vi "Build-timeline.vi"(8 "error in (no error)":errorcluster, 10 "Temp-timeline in":T1={"Previous point"={"Start time [µs]"=0, "End time [µs]"=0, "X [mm]"=0.0, "Y [mm]"=0.0, "Type"=enum."BeginJob", "Speed [mm/µs]"=0.0, "Direction [rad]"=0.0, "X [bit]"=0, "Y [bit]"=0, "Speed [bit/µs]"=0.0, "Power [W]"=0.0, "Power [bit]"=0, "JumpDelay"=0, "MarkDelay"=0, "PolyDelay"=0, "LaserOnDelay"=0, "LaserOffDelay"=0, "LaserPowerDelay"=0, "LaserEnableDelay"=0, "Xraw [mm]"=0.0, "Yraw [mm]"=0.0}, "Current point"={"Start time [µs]"=0, "End time [µs]"=0, "X [mm]"=0.0, "Y [mm]"=0.0, "Type"=enum."BeginJob", "Speed [mm/µs]"=0.0, "Direction [rad]"=0.0, "X [bit]"=0, "Y [bit]"=0, "Speed [bit/µs]"=0.0, "Power [W]"=0.0, "Power [bit]"=0, "JumpDelay"=0, "MarkDelay"=0, "PolyDelay"=0, "LaserOnDelay"=0, "LaserOffDelay"=0, "LaserPowerDelay"=0, "LaserEnableDelay"=0, "Xraw [mm]"=0.0, "Yraw [mm]"=0.0}, "Path"=[], "Current properties"={"ItemID"=0, "Start time"=0, "EffectiveOffset"=[0.0, 0.0], "EffectiveTranfsorm"=[[1.0, 0.0], [0.0, 1.0]], "Z-Offset"=0.0, "Units"=enum."mm", "LaserPower"=0, "Started"=FALSE, "Enabled"=FALSE, "FieldOffset"=[0.0, 0.0], "Offset"=[0.0, 0.0], "TransformEnable"=TRUE, "XYCalFactor"=196.0, "JumpSpeed"={"unit/us"=0.0, "Tick interval us"=0, "Bits per interval"=0}, "MarkSpeed"={"unit/us"=0.0, "Tick interval us"=0, "Bits per interval"=0}}}, 11 "Element-XML in":refnum<class "BeginJob.lvclass">) -> (0 "error out":errorcluster, 2 "Temp-timeline":T1={"Previous point"={"Start time [µs]"=0, "End time [µs]"=0, "X [mm]"=0.0, "Y [mm]"=0.0, "Type"=enum."BeginJob", "Speed [mm/µs]"=0.0, "Direction [rad]"=0.0, "X [bit]"=0, "Y [bit]"=0, "Speed [bit/µs]"=0.0, "Power [W]"=0.0, "Power [bit]"=0, "JumpDelay"=0, "MarkDelay"=0, "PolyDelay"=0, "LaserOnDelay"=0, "LaserOffDelay"=0, "LaserPowerDelay"=0, "LaserEnableDelay"=0, "Xraw [mm]"=0.0, "Yraw [mm]"=0.0}, "Current point"={"Start time [µs]"=0, "End time [µs]"=0, "X [mm]"=0.0, "Y [mm]"=0.0, "Type"=enum."BeginJob", "Speed [mm/µs]"=0.0, "Direction [rad]"=0.0, "X [bit]"=0, "Y [bit]"=0, "Speed [bit/µs]"=0.0, "Power [W]"=0.0, "Power [bit]"=0, "JumpDelay"=0, "MarkDelay"=0, "PolyDelay"=0, "LaserOnDelay"=0, "LaserOffDelay"=0, "LaserPowerDelay"=0, "LaserEnableDelay"=0, "Xraw [mm]"=0.0, "Yraw [mm]"=0.0}, "Path"=[], "Current properties"={"ItemID"=0, "Start time"=0, "EffectiveOffset"=[0.0, 0.0], "EffectiveTranfsorm"=[[1.0, 0.0], [0.0, 1.0]], "Z-Offset"=0.0, "Units"=enum."mm", "LaserPower"=0, "Started"=FALSE, "Enabled"=FALSE, "FieldOffset"=[0.0, 0.0], "Offset"=[0.0, 0.0], "TransformEnable"=TRUE, "XYCalFactor"=196.0, "JumpSpeed"={"unit/us"=0.0, "Tick interval us"=0, "Bits per interval"=0}, "MarkSpeed"={"unit/us"=0.0, "Tick interval us"=0, "Bits per interval"=0}}}, 3 "Element-XML out":refnum<class "BeginJob.lvclass">)   [LabVIEW 2013, in "MaterialCharacterization.lvlib" / "BeginJob.lvclass"]
uses:
  BeginJob.lvclass
  ScanParser/Path-buffer.ctl
  ScanParser/Point-buffer.ctl
  Elements.ctl
  ScanParser/Property-buffer.ctl
  ScanParser/Units.ctl
  ScanParser/Speed.ctl
  Element-XML.lvclass
  ScanParser/MC-ScanParser.lvclass
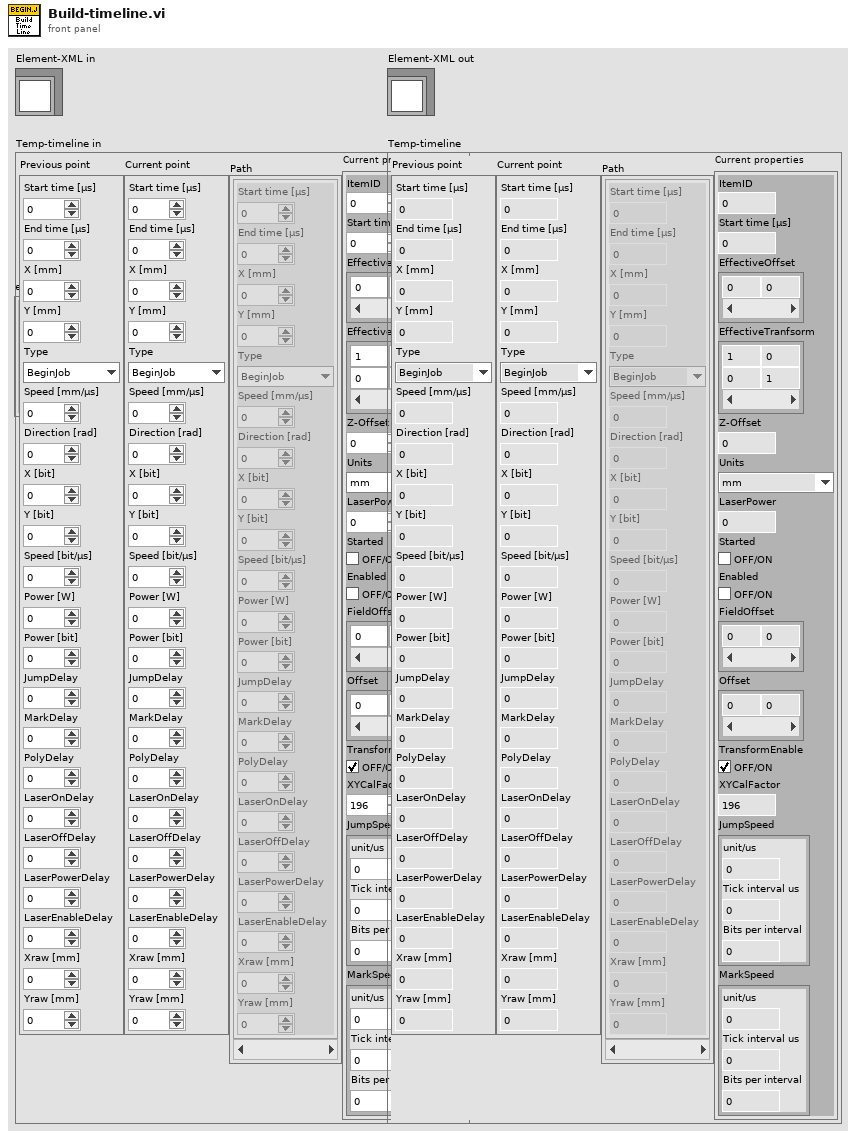
[diagram p1: front panel]
types:
  T1 = typedef "MaterialCharacterization.lvlib/MC-ScanParser.lvclass/Path-buffer.ctl" = cluster{"Previous point":T2, "Current point":T2, "Path":T2[], "Current properties":T4}
  T2 = typedef "MaterialCharacterization.lvlib/MC-ScanParser.lvclass/Point-buffer.ctl" = cluster{"Start time [µs]":i64, "End time [µs]":i64, "X [mm]":dbl, "Y [mm]":dbl, "Type":T3, "Speed [mm/µs]":dbl, "Direction [rad]":dbl, "X [bit]":i16, "Y [bit]":i16, "Speed [bit/µs]":dbl, "Power [W]":dbl, "Power [bit]":u8, "JumpDelay":i64, "MarkDelay":i64, "PolyDelay":i64, "LaserOnDelay":i64, "LaserOffDelay":i64, "LaserPowerDelay":i64, "LaserEnableDelay":i64, "Xraw [mm]":dbl, "Yraw [mm]":dbl}
  T3 = typedef "MaterialCharacterization.lvlib/Element-XML.lvclass/Elements.ctl" = enum16{"BeginJob", "WriteDigital", "WriteAnalog", "Set", "ApplicationEvent", "JumpAbs", "MarkAbs", "JumpRel", "MarkRel", "LongDelay", "EndJob"}
  T4 = typedef "MaterialCharacterization.lvlib/MC-ScanParser.lvclass/Property-buffer.ctl" = cluster{"ItemID":u32, "Start time":i64, "EffectiveOffset":dbl[], "EffectiveTranfsorm":dbl[][], "Z-Offset":sgl, "Units":T5, "LaserPower":u8, "Started":bool, "Enabled":bool, "FieldOffset":dbl[], "Offset":dbl[], "TransformEnable":bool, "XYCalFactor":dbl, "JumpSpeed":T6, "MarkSpeed":T6}
  T5 = typedef "MaterialCharacterization.lvlib/MC-ScanParser.lvclass/Units.ctl" = enum16{"bits", "mm", "inch", "mils"}
  T6 = typedef "MaterialCharacterization.lvlib/MC-ScanParser.lvclass/Speed.ctl" = cluster{"unit/us":dbl, "Tick interval us":u16, "Bits per interval":u16}
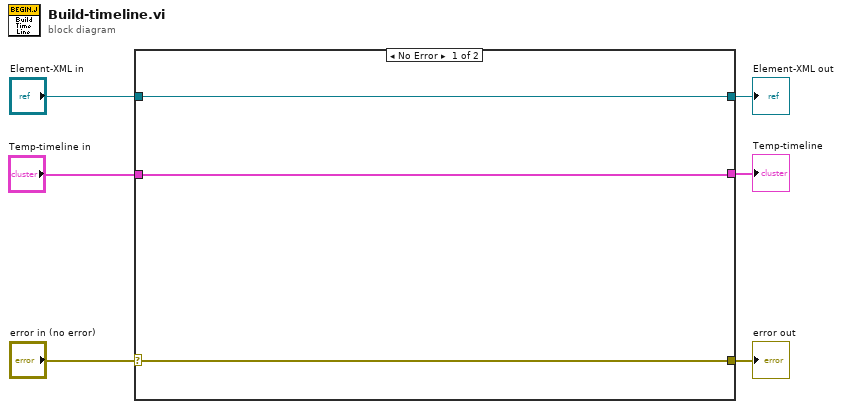
[diagram p0: block diagram]
diagram:
  n1 = case shown="No Error" "error in (no error)" {
    selector: "error in (no error)" -> [w8 w12]
    tunnel: [w8 w12] -> w5
    tunnel: [w9 w11] -> w3
    tunnel: "Element-XML in" -> [w9 w11]
    tunnel: "Temp-timeline in" -> [w7 w10]
    tunnel: [w7 w10] -> w1
    frame No Error {
    }
    frame Error {
    }
  }
  "error out" <- w5
  "Element-XML out" <- w3
  "Temp-timeline" <- w1
